vi "CreateUnaryOperator.vi"(5 "UnaryOperator In":refnum<class "UnaryOperator.lvclass">, 8 "error in (no error)":errorcluster, 10 "Constraint":refnum<class "Constraint.lvclass">) -> (0 "error out":errorcluster, 3 "UnaryOperator":refnum<class "UnaryOperator.lvclass">)   [LabVIEW 2019, in "Constraint.lvlib" / "UnaryOperator.lvclass"]
uses:
  UnaryOperator.lvclass
  Constraint/Constraint.lvclass
  UnaryOperator.lvclass/UnaryOperator.ctl
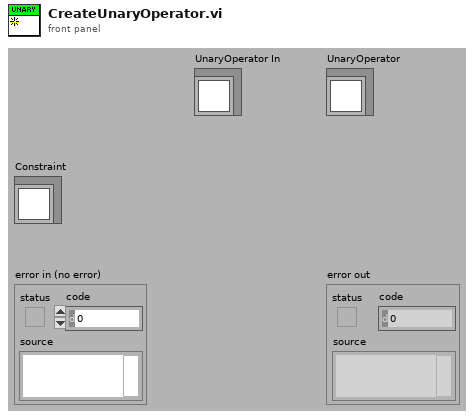
[diagram p1: front panel]
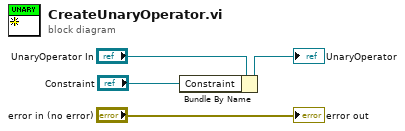
[diagram p0: block diagram]
diagram:
  n1 = Bundle By Name(cluster="UnaryOperator In", "Constraint"="Constraint") -> (→"UnaryOperator":refnum<class "UnaryOperator.lvclass">)
  "error out" <- "error in (no error)"
